vi "Uart read.vi"(0 "RedPitaya connection in":refnum<k5>, 3 "timeout ms (2000)":i32=2000, 11 "error in":errorcluster) -> (4 "RedPitaya connection out":refnum<k5>, 6 "data out":string, 15 "error out":errorcluster)   [LabVIEW 2021]
uses:
  Red Pitaya Labview Lib/Red_Pitaya_LabVIEW_Driver&Examples/Red_Pitaya/RedPitaya.lvlib
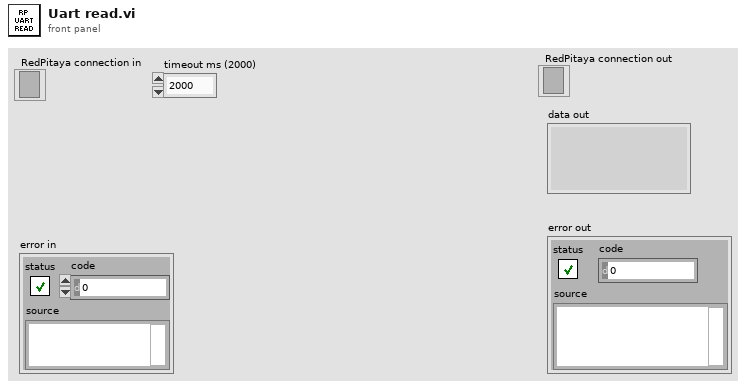
[diagram p1: front panel]
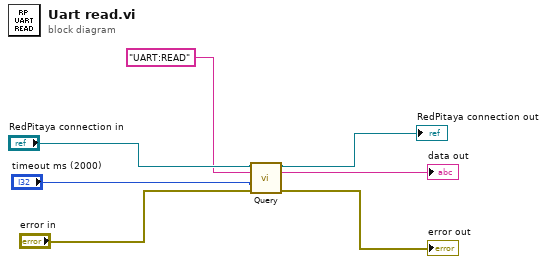
[diagram p0: block diagram]
diagram:
  n1 = call "Query.vi"("RedPitaya connection in"="RedPitaya connection in", "SCPI Query"="UART:READ", "timeout ms (2000)"="timeout ms (2000)", "error in"="error in") -> ("RedPitaya connection out"=→"RedPitaya connection out":refnum<k5>, "data out"=→"data out":string, "error out"=→"error out":errorcluster)  [unwired: 9 in]
